vi "StateSpaceVectorComputeVI.vi"(0 "Mass of Bottom Wheel (M)":dbl, 1 "Mass of Rest (m)":dbl, 2 "Kinetic friction of robot (b)":dbl, 3 "Length to center of mass (l)":dbl, 4 "Inertia of pendulum (I)":dbl) -> (5 "A":dbl[][](array[numeric]), 6 "B":dbl[][](array[numeric]), 7 "C":dbl[][](array[numeric]), 8 "D":dbl[][](array[numeric]))   [LabVIEW 2012]
uses:
  <vilib>/imath/engines/lvmath2/RunTimeEngine/ErrorHandling/NIMS_Finalize Error.vi
  <vilib>/imath/engines/lvmath2/RunTimeEngine/NodeEndStatement/NIMS_NodeEndStatement_Output.vi
  <instcachedir>/0/NIMS_NodeEndStatement_Output_53EC0D466D134D7ABD903AC30B43404B.lvgen/NIMS_NodeEndStatement_Output_53EC0D466D134D7ABD903AC30B43404B_002.vi
  <vilib>/imath/engines/lvmath2/RunTimeEngine/ReplaceToken/NIMS_Replace - Check Row.vi
  <instcachedir>/0/NIMS_Replace - Check Row_8C35B66FE73A429EAC382AAA935851F0.lvgen/NIMS_Replace - Check Row_8C35B66FE73A429EAC382AAA935851F0_005.vi
  <vilib>/imath/engines/lvmath2/RunTimeEngine/ReplaceToken/NIMS_Replace - Check Column.vi
  <instcachedir>/0/NIMS_Replace - Check Column_F9ADE87E459D46779ACFAE3AFB317B9B.lvgen/NIMS_Replace - Check Column_F9ADE87E459D46779ACFAE3AFB317B9B_007.vi
  <vilib>/imath/engines/lvmath2/RunTimeEngine/ReplaceToken/NIMS_Replace - Size Check M(_,_)=S.vi
  <instcachedir>/0/NIMS_Replace - Size Check M(_,_)=S_0CFA00F12BB840EDA61E43D782562782.lvgen/NIMS_Replace - Size Check M(_,_)=S_0CFA00F12BB840EDA61E43D782562782_002.vi
  <vilib>/imath/engines/lvmath2/RunTimeEngine/ReplaceToken/NIMS_Replace - M(S,S)=S.vi
  <instcachedir>/0/NIMS_Replace - M(S,S)=S_59120E3D3E804D63A1B2B7FDD4B95F55.lvgen/NIMS_Replace - M(S,S)=S_59120E3D3E804D63A1B2B7FDD4B95F55_002.vi
  <vilib>/imathl/engines/lvmath/Functions/Error Handling/Create Error.vi
  <instcachedir>/0/NIMS_Replace - Check Row_8C35B66FE73A429EAC382AAA935851F0.lvgen/NIMS_Replace - Check Row_8C35B66FE73A429EAC382AAA935851F0_000.vi
  <instcachedir>/0/NIMS_Replace - Check Column_F9ADE87E459D46779ACFAE3AFB317B9B.lvgen/NIMS_Replace - Check Column_F9ADE87E459D46779ACFAE3AFB317B9B_001.vi
  <instcachedir>/0/NIMS_Replace - Size Check M(_,_)=S_0CFA00F12BB840EDA61E43D782562782.lvgen/NIMS_Replace - Size Check M(_,_)=S_0CFA00F12BB840EDA61E43D782562782_000.vi
  <instcachedir>/0/NIMS_Replace - M(S,S)=S_59120E3D3E804D63A1B2B7FDD4B95F55.lvgen/NIMS_Replace - M(S,S)=S_59120E3D3E804D63A1B2B7FDD4B95F55_000.vi
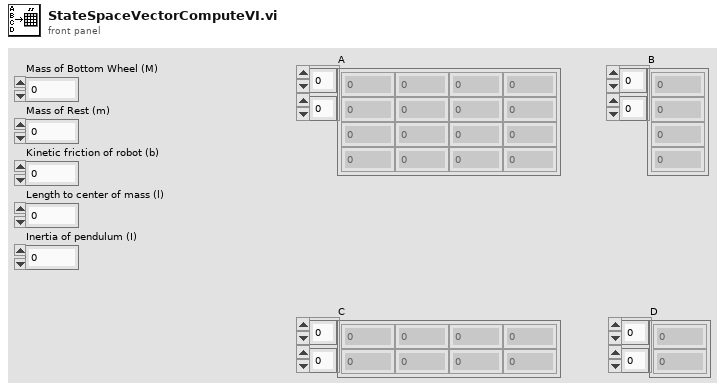
[diagram p1: front panel]
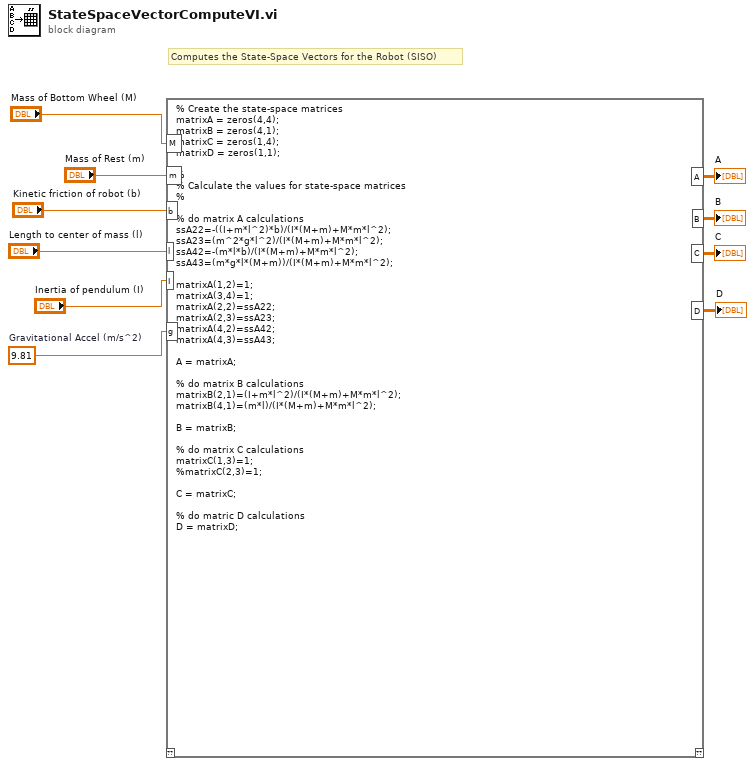
[diagram p0: block diagram]
diagram:
  w5 = 9.81  # Gravitational Accel (m/s^2)
  # "Computes the State-Space Vectors for the Robot (SISO)"
  n1 = mathscript code="% Create the state-space matrices\nmatrixA = zeros(4,4);\nmatrixB = zeros(4,1);\nmatrixC = zeros(1,4);\nmatrixD = zeros(1,1);\n\n%\n% Calculate the values for state-space matrices\n%\n\n% do matrix A calculations\nssA22=-((I+m*l^2)*b)/(I*(M+m)+M*m*l^2);\nssA23=(m^2*g*l^2)/(I*(M+m)+M*m*l^2);\nssA42=-(m*l*b)/(I*(M+m)+M*m*l^2);\nssA43=(m*g*l*(M+m))/(I*(M+m)+M*m*l^2);\n\nmatrixA(1,2)=1;\nmatrixA(3,4)=1;\nmatrixA(2,2)=ssA22;\nmatrixA(2,3)=ssA23;\nmatrixA(4,2)=ssA42;\nmatrixA(4,3)=ssA43;\n\nA = matrixA;\n\n% do matrix B calculations\nmatrixB(2,1)=(I+m*l^2)/(I*(M+m)+M*m*l^2);\nmatrixB(4,1)=(m*l)/(I*(M+m)+M*m*l^2);\n\nB = matrixB;\n\n% do matrix C calculations\nmatrixC(1,3)=1;\n%matrixC(2,3)=1;\n\nC = matrixC;\n\n% do matric D calculations\nD = matrixD;"("M"="Mass of Bottom Wheel (M)", "m"="Mass of Rest (m)", "b"="Kinetic friction of robot (b)", "l"="Length to center of mass (l)", "I"="Inertia of pendulum (I)", "g"=w5) -> ("A"=→"A":dbl[][], "B"=→"B":dbl[][], "D"=→"D":dbl[][], "C"=→"C":dbl[][])  [unwired: 1 in, 1 out]
